vi "Get All Property.vi"(8 "error in":errorcluster, 11 "Item Ref in":refnum<data-value>) -> (0 "error out":errorcluster, 3 "Properties Ref out":refnum<data-value>[](array[refnum]))   [LabVIEW 2024, in "Config File Parser.lvlib" / "Property.lvclass"]
uses:
  Property.lvclass
  Property.lvclass/Property.ctl
  Item/Item.lvclass
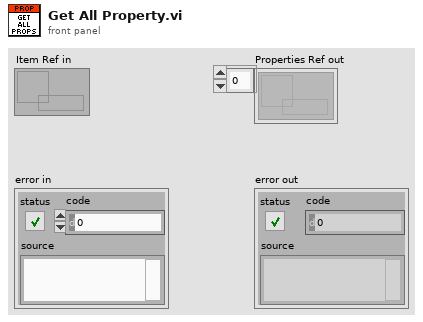
[diagram p1: front panel]
types:
  T1 = typedef "Config File Parser.lvlib/Item.lvclass/Item Type.ctl" = enum16{"Property", "Channel", "Section"}
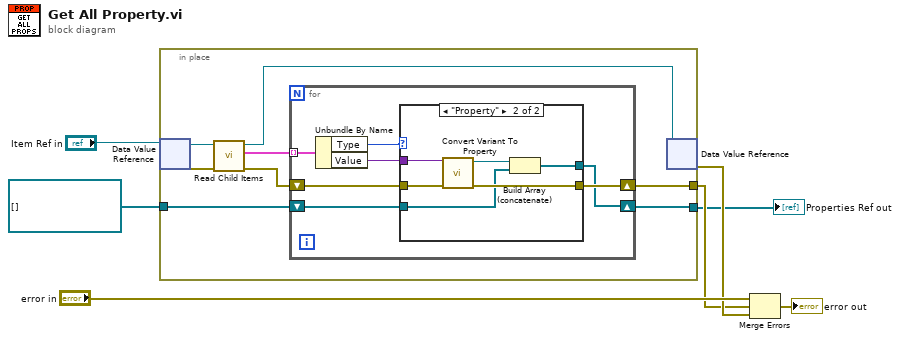
[diagram p0: block diagram]
diagram:
  n1 = in-place {
    in-place-border: refnum<data-value>[] [] -> [w10]
    in-place-border: [w8] -> w1
    in-place-border: [w13] -> w4
    n2 = in-place-dvr #1("Item Ref in") -> (w12:refnum<class "Item.lvclass">, w15:errorcluster)
    n3 = call-dynamic "Read Child Items.vi"("error in"=w15, "Item in"=w12) -> ("error out"=w14:errorcluster, "Child Items"=w11:cluster{"Type":T1, "Value":variant}[], "Item out"=w9:refnum<class "Item.lvclass">)  [unwired: 7 in]
    n4 = for {
      tunnel: w11 -> [w20] mode=indexing
      shift-right: [w16] -> w8
      shift-left: w10 -> [w17]
      shift-right: [w21] -> w13
      shift-left: w14 -> [w22]
      n5 = Unbundle By Name(w20) -> ("Type"=w19:T1, "Value"=w18:variant)
      n6 = case shown="\"Property\"" w19 {
        tunnel: w18 -> [_ w28]
        tunnel: w17 -> [w23 w26]
        tunnel: [w23 w25] -> w16
        tunnel: w22 -> [w24 w30]
        tunnel: [w24 w29] -> w21
        frame Default {
        }
        frame "Property" {
          n7 = call "Convert Variant To Property.vi"("error in"=w30, "Property Variant"=w28) -> ("error out"=w29:errorcluster, "Property Ref out"=w27:refnum<data-value>)  [unwired: 8 in]
          n8 = Build Array (concatenate)(w27, w26) -> (w25:refnum<data-value>[])
        }
      }
    }
    n9 = in-place-dvr #1(w9) -> (w6:errorcluster)  [unwired: 1 out]
  }
  "Properties Ref out" <- w1
  n10 = Merge Errors("error in", w4, w6) -> (→"error out":errorcluster)
